vi "Blob____Center.vi"(7 "ROI":T3, 8 "error in (no error)":errorcluster, 9 "Edge Strength Cluster":cluster{"Lower value":sgl, "Upper value":sgl}={"Lower value"=50.0, "Upper value"=255.0}, 10 "Area Limits Cluster":T1={"Area Lower Value"=2000.0, "Area Upper Value"=12000.0} {"Area Upper Value" format="%#_13g"}, 11 "Image Out":T2(plugin-control)) -> (0 "error out":errorcluster, 3 "Co Ordinate System":T4)   [LabVIEW 2019, in "Algorithm.lvclass"]
uses:
  FrameworkOverrides/Algorithm.lvclass
  <vilib>/vision/NI_Vision_Development_Module.lvlib
panel:
  out "element":dbl
  out "Particle Measurements (Pixels)":dbl[][](array[numeric]) format="%.2f"
  out "Area":dbl[](array[numeric])
  out "Image Out (duplicate)":T2(plugin-control)
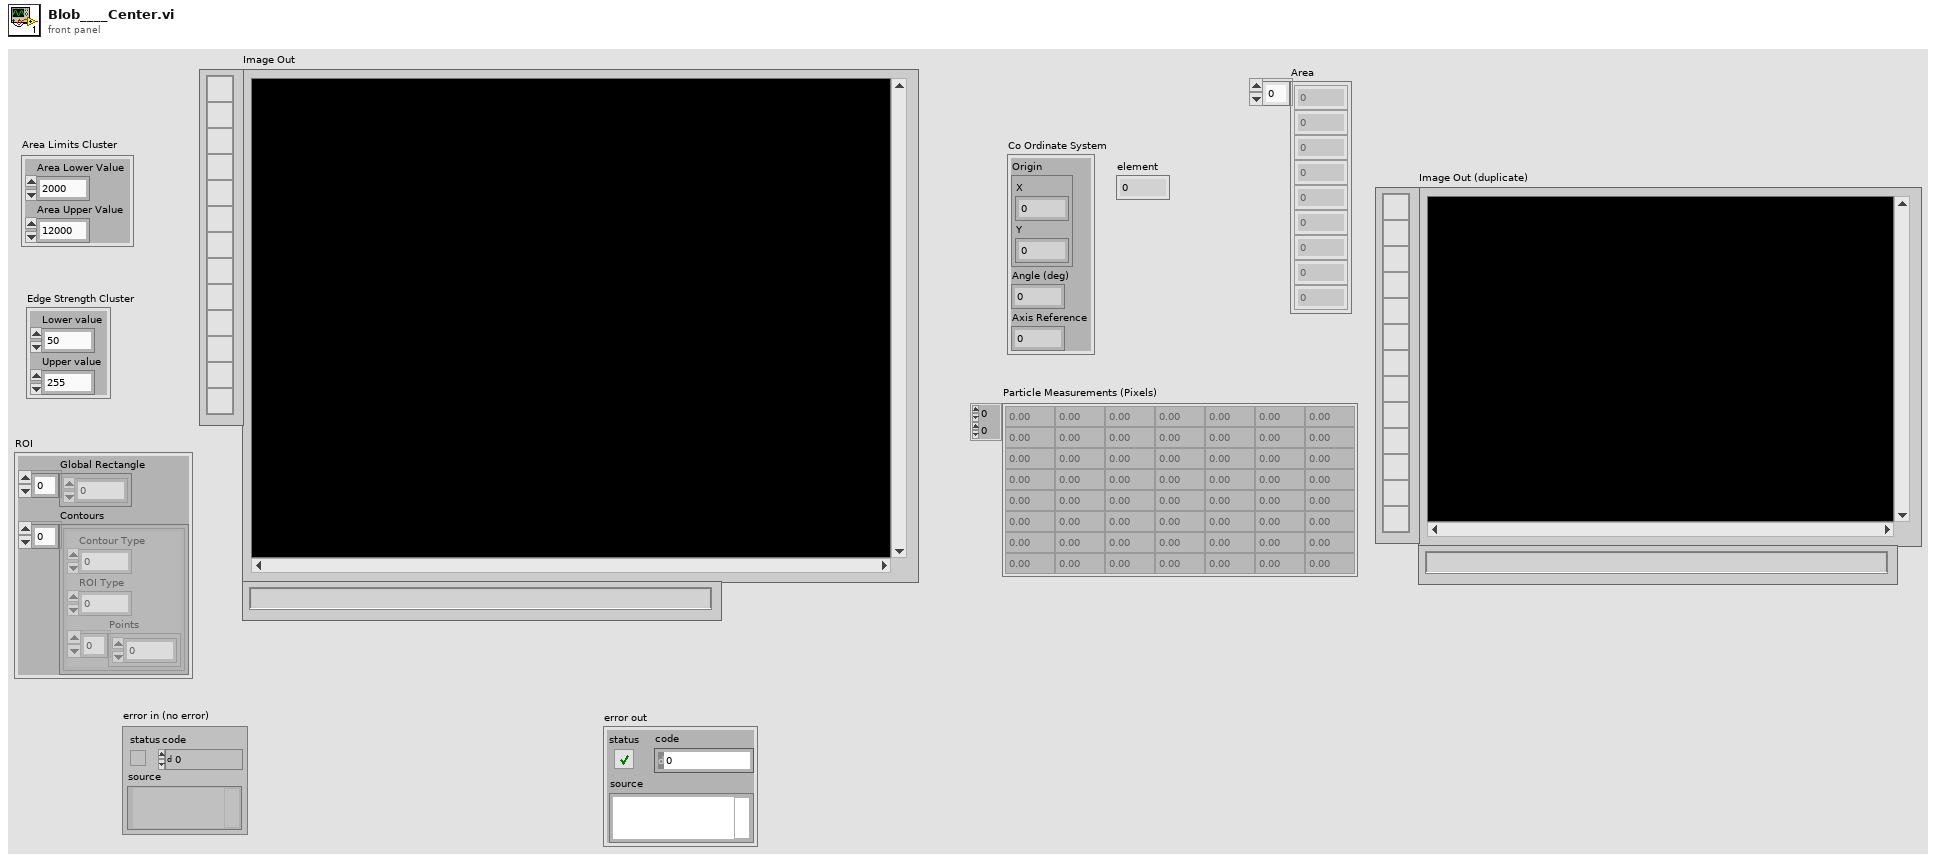
[diagram p1: front panel]
types:
  T1 = cluster{"Area Lower Value":dbl, "Area Upper Value":dbl}
  T2 = typedef "IMAQ Image.ctl" = refnum<image>
  T3 = cluster{"Global Rectangle":i32[], "Contours":cluster{"Contour Type":u32, "ROI Type":u32, "Points":i32[]}[]}
  T4 = cluster{"Origin":cluster{"X":sgl, "Y":sgl}, "Angle (deg)":sgl, "Axis Reference":u32}
  T5 = typedef "Particle Parameters" = i32
  T6 = cluster{"Measurement Parameter":T5, "Range Lower Value":dbl, "Range Upper Value":dbl, "Range":bool, "Measurement Type":bool}
  T7 = typedef "Image Type" = u32
  T8 = cluster{"Measurement Parameter":T5, "Range Lower Value":dbl, "Range Upper Value":dbl, "Range":bool, "Measurement Type":bool}[]
  T9 = typedef "IMAQ Rectangle" = cluster{"Left":i32, "Top":i32, "Right":i32, "Bottom":i32, "Rotation":dbl}
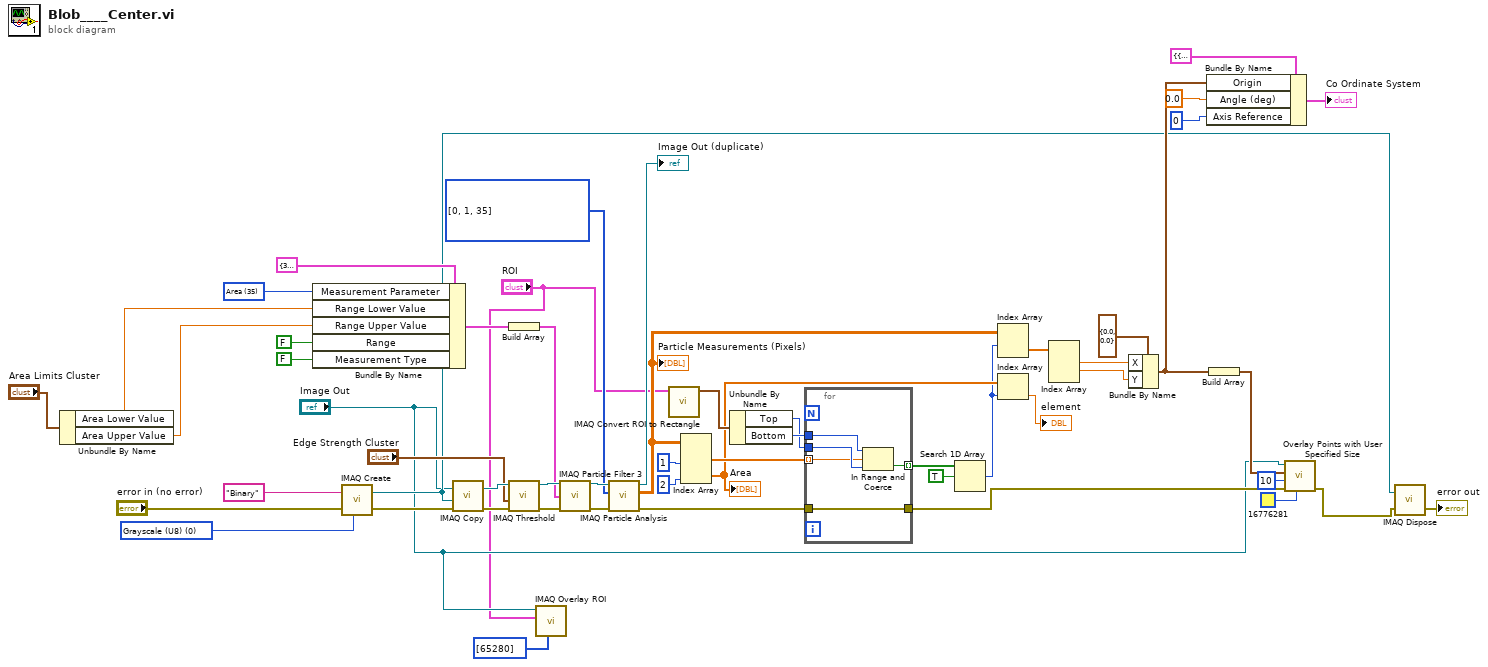
[diagram p0: block diagram]
diagram:
  w21 = T5[] [0, 1, 35] items=["Center of Mass X", "Center of Mass Y", "First Pixel X", "First Pixel Y", "Bounding Rect Left", "Bounding Rect Top", "Bounding Rect Right", "Bounding Rect Bottom", "Max Feret Diameter Start X", "Max Feret Diameter Start Y", "Max Feret Diameter End X", "Max Feret Diameter End Y", "Max Horiz. Segment Length Left", "Max Horiz. Segment Length Right", "Max Horiz. Segment Length Row", "-", "Bounding Rect Width", "Bounding Rect Height", "Bounding Rect Diagonal", "Perimeter", "Convex Hull Perimeter", "Holes' Perimeter", "Max Feret Diameter", "Equivalent Ellipse Major Axis", "Equivalent Ellipse Minor Axis", "Equivalent Ellipse Minor Axis (Feret)", "Equivalent Rect Long Side", "Equivalent Rect Short Side", "Equivalent Rect Diagonal", "Equivalent Rect Short Side (Feret)", "Average Horiz. Segment Length", "Average Vert. Segment Length", "Hydraulic Radius", "Waddel Disk Diameter", "-", "Area", "Holes' Area", "Particle & Holes' Area", "Convex Hull Area", "Image Area", "-", "Number of Holes", "Number of Horiz. Segments", "Number of Vert. Segments", "-", "Orientation", "Max Feret Diameter Orientation", "-", "% Area/Image Area", "% Area/(Particle & Holes' Area)", "Ratio of Equivalent Ellipse Axes", "Ratio of Equivalent Rect Sides", "-", "Elongation Factor", "Compactness Factor", "Heywood Circularity Factor", "Type Factor", "-", "Sum X", "Sum Y", "Sum XX", "Sum XY", "Sum YY", "Sum XXX", "Sum XXY", "Sum XYY", "Sum YYY", "-", "Moment of Inertia XX", "Moment of Inertia XY", "Moment of Inertia YY", "Moment of Inertia XXX", "Moment of Inertia XXY", "Moment of Inertia XYY", "Moment of Inertia YYY", "Norm. Moment of Inertia XX", "Norm. Moment of Inertia XY", "Norm. Moment of Inertia YY", "Norm. Moment of Inertia XXX", "Norm. Moment of Inertia XXY", "Norm. Moment of Inertia XYY", "Norm. Moment of Inertia YYY", "Hu Moment 1", "Hu Moment 2", "Hu Moment 3", "Hu Moment 4", "Hu Moment 5", "Hu Moment 6", "Hu Moment 7"] ("Pixel Measurements")
  w38 = T5 35 items=["Center of Mass X", "Center of Mass Y", "First Pixel X", "First Pixel Y", "Bounding Rect Left", "Bounding Rect Top", "Bounding Rect Right", "Bounding Rect Bottom", "Max Feret Diameter Start X", "Max Feret Diameter Start Y", "Max Feret Diameter End X", "Max Feret Diameter End Y", "Max Horiz. Segment Length Left", "Max Horiz. Segment Length Right", "Max Horiz. Segment Length Row", "-", "Bounding Rect Width", "Bounding Rect Height", "Bounding Rect Diagonal", "Perimeter", "Convex Hull Perimeter", "Holes' Perimeter", "Max Feret Diameter", "Equivalent Ellipse Major Axis", "Equivalent Ellipse Minor Axis", "Equivalent Ellipse Minor Axis (Feret)", "Equivalent Rect Long Side", "Equivalent Rect Short Side", "Equivalent Rect Diagonal", "Equivalent Rect Short Side (Feret)", "Average Horiz. Segment Length", "Average Vert. Segment Length", "Hydraulic Radius", "Waddel Disk Diameter", "-", "Area", "Holes' Area", "Particle & Holes' Area", "Convex Hull Area", "Image Area", "-", "Number of Holes", "Number of Horiz. Segments", "Number of Vert. Segments", "-", "Orientation", "Max Feret Diameter Orientation", "-", "% Area/Image Area", "% Area/(Particle & Holes' Area)", "Ratio of Equivalent Ellipse Axes", "Ratio of Equivalent Rect Sides", "-", "Elongation Factor", "Compactness Factor", "Heywood Circularity Factor", "Type Factor", "-", "Sum X", "Sum Y", "Sum XX", "Sum XY", "Sum YY", "Sum XXX", "Sum XXY", "Sum XYY", "Sum YYY", "-", "Moment of Inertia XX", "Moment of Inertia XY", "Moment of Inertia YY", "Moment of Inertia XXX", "Moment of Inertia XXY", "Moment of Inertia XYY", "Moment of Inertia YYY", "Norm. Moment of Inertia XX", "Norm. Moment of Inertia XY", "Norm. Moment of Inertia YY", "Norm. Moment of Inertia XXX", "Norm. Moment of Inertia XXY", "Norm. Moment of Inertia XYY", "Norm. Moment of Inertia YYY", "Hu Moment 1", "Hu Moment 2", "Hu Moment 3", "Hu Moment 4", "Hu Moment 5", "Hu Moment 6", "Hu Moment 7"] ("Measurement Parameter")
  w51 = T7 0 items=["Grayscale (U8)", "Grayscale (I16)", "Grayscale (SGL)", "Complex (CSG)", "RGB (U32)", "HSL (U32)", "RGB (U64)", "Grayscale (U16)"] ("Image Type")
  n1 = Unbundle By Name("Area Limits Cluster") -> ("Area Lower Value"=w11:dbl, "Area Upper Value"=w10:dbl)
  n2 = Bundle By Name(cluster=T6 {"Measurement Parameter"=35, "Range Lower Value"=16000.0, "Range Upper Value"=25000.0, "Range"=FALSE, "Measurement Type"=FALSE} ("Selection Value"), "Measurement Parameter"=w38, "Range Lower Value"=w11, "Range Upper Value"=w10, "Range"=FALSE, "Measurement Type"=FALSE) -> (w37:T6)
  n3 = call "IMAQ Create"("Image Name"="Binary", "Image Type"=w51, "error in (no error)"="error in (no error)") -> ("New Image"=w9:T2, "error out"=w47:errorcluster)  [unwired: 2 in]
  n4 = call "IMAQ Copy"("error in (no error)"=w47, "Image Dst"=w9, "Image Src"="Image Out") -> ("error out"=w34:errorcluster, "Image Dst Out"=w54:T2)  [unwired: 3 in]
  n5 = Build Array(w37) -> (w36:T8)
  n6 = call "IMAQ Threshold"("error in (no error)"=w34, "Range"="Edge Strength Cluster", "Image Src"=w54) -> ("error out"=w30:errorcluster, "Image Dst Out"=w49:T2)  [unwired: 7 in]
  n7 = call "IMAQ Overlay ROI"("Colors (Green)"=u32[] [65280], "ROI Descriptor"="ROI", "Image"="Image Out") -> ()  [unwired: 7 in, 2 out]
  n8 = call "IMAQ Particle Filter 3"("Image Src"=w49, "Selection Values"=w36, "error in (no error)"=w30) -> ("Image Dst Out"=w52:T2, "error out"=w53:errorcluster)  [unwired: 10 in, 1 out]
  n9 = call "IMAQ Particle Analysis"("error in (no error)"=w53, "Pixel Measurements"=w21, "Image"=w52) -> ("error out"=w29:errorcluster, "Particle Measurements (Pixels)"=w25:dbl[][], "Image Out (duplicate)"=→"Image Out (duplicate)":T2)  [unwired: 3 in, 3 out]
  "Particle Measurements (Pixels)" <- w25
  n10 = call "IMAQ Convert ROI to Rectangle"("ROI Descriptor"="ROI") -> ("Rectangle"=w33:T9)  [unwired: 8 in, 1 out]
  n11 = Index Array(array=w25, index (col) #1=1 ("disabled index (col)"), index (col) #2=2 ("index (col)")) -> (element #1=w20:dbl[], element #2=w17:dbl[])  [unwired: 2 in]
  "Area" <- w17
  n12 = Unbundle By Name(w33) -> ("Top"=w31:i32, "Bottom"=w32:i32)
  n13 = for {
    tunnel: w32 -> [w59]
    tunnel: w31 -> [w58]
    tunnel: w29 -> [w57]
    tunnel: [w57] -> w8
    tunnel: [w55] -> w27 mode=indexing
    tunnel: w20 -> [w56] mode=indexing
    n14 = In Range and Coerce(upper limit=w59, x=w56, lower limit=w58) -> (In Range?=w55:bool)  [unwired: 1 out]
  }
  n15 = Search 1D Array(1D array=w27, element=TRUE) -> (index of element=w16:i32)  [unwired: 1 in]
  n16 = Index Array(array=w25, index (row)=w16) -> (element=w24:dbl[])  [unwired: 1 in]
  n17 = Index Array(array=w17, index=w16) -> (element=→"element":dbl)
  n18 = Index Array(array=w24) -> (element #1=w23:dbl, element #2=w22:dbl)  [unwired: 3 in, 1 out]
  n19 = Bundle By Name(cluster=cluster{"X":sgl, "Y":sgl} {"X"=0.0, "Y"=0.0} ("Origin"), "X"=w23, "Y"=w22) -> (w42:cluster{"X":sgl, "Y":sgl})
  n20 = Bundle By Name(cluster=T4 {"Origin"={"X"=0.0, "Y"=0.0}, "Angle (deg)"=0.0, "Axis Reference"=0} ("Coordinate System"), "Origin"=w42, "Angle (deg)"=sgl 0.0, "Axis Reference"=u32 0) -> (→"Co Ordinate System":T4)
  n21 = Build Array(w42) -> (w6:cluster{"X":sgl, "Y":sgl}[])
  n22 = call "Overlay Points with User Specified Size.vi"("Color"=u32 16776281, "error in"=w8, "Point Diameter (5)"=u32 10, "Points"=w6, "Image In"="Image Out") -> ("error out"=w7:errorcluster)  [unwired: 5 in, 1 out]
  n23 = call "IMAQ Dispose"("Image"=w9, "error in (no error)"=w7) -> ("error out"=→"error out":errorcluster)  [unwired: 4 in]
